vi "Station jsObject Array.vi"(6 "Stations Instruments (none)":cluster{"Instruments":T1[]}[](array[cluster]), 8 "error in (no error)":errorcluster, 9 "Stations (empty)":T2[](array[typedef]), 10 "Stations jsObject Array Name (\"STATIONS\")":string="STATIONS", 11 "Previous String (\"\")":string) -> (0 "error out":errorcluster, 2 "Stations jsObject Array":string, 3 "Station jsObject Definition":string)   [LabVIEW 2011]
uses:
  Station Record.ctl
  Instruments/Instrument Record.ctl
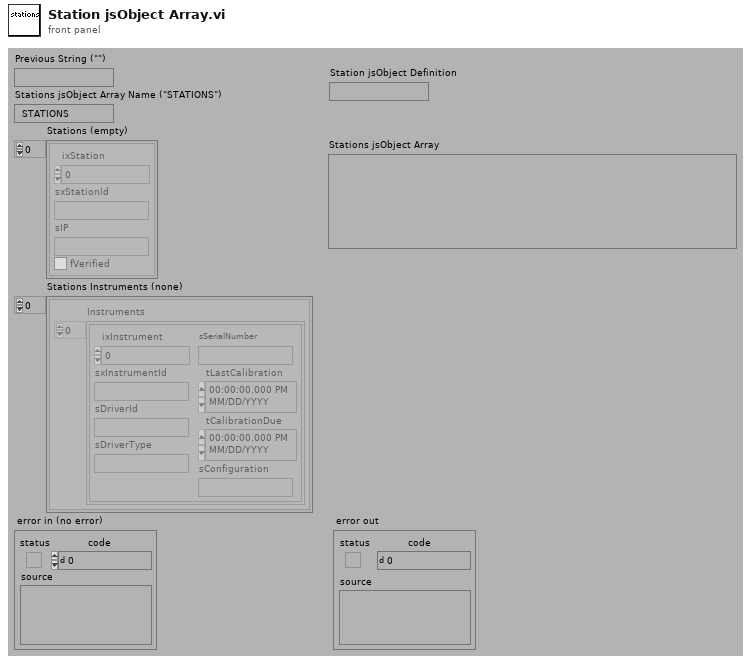
[diagram p1: front panel]
types:
  T1 = typedef "Instrument Record.ctl" = cluster{"ixInstrument":i32, "sxInstrumentId":string, "sDriverId":string, "sDriverType":string, "sSerialNumber":string, "tLastCalibration":timestamp, "tCalibrationDue":timestamp, "sConfiguration":string}
  T2 = typedef "Station Record.ctl" = cluster{"ixStation":i32, "sxStationId":string, "sIP":string, "fVerified":bool}
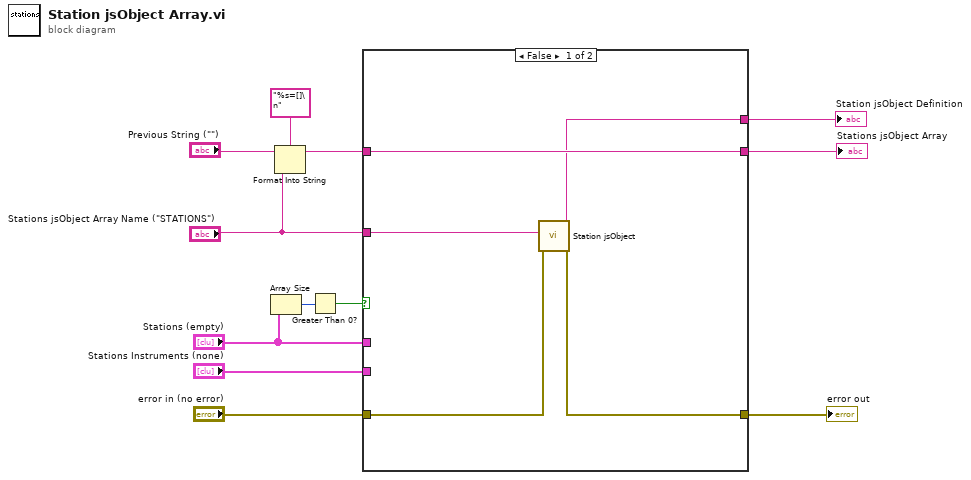
[diagram p0: block diagram]
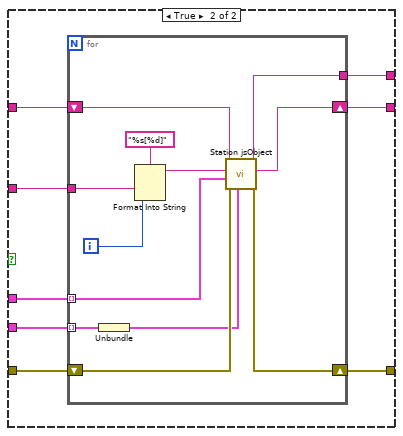
[diagram p2: hidden frame]
diagram:
  n1 = Array Size(array="Stations (empty)") -> (size(s)=w10:i32)
  n2 = Format Into String(format string="%s=[]\n", initial string="Previous String (\"\")", "Stations jsObject Array Name (\"STATIONS\")") -> (resulting string=w11:string)  [unwired: 1 in, 1 out]
  n3 = Greater Than 0?(x=w10) -> (x > 0?=w9:bool)
  n4 = case shown="False" w9 {
    tunnel: w11 -> [w17 w25]
    tunnel: "error in (no error)" -> [w16 w24]
    tunnel: [w17 w23] -> w3
    tunnel: [w15 w22] -> w2
    tunnel: "Stations jsObject Array Name (\"STATIONS\")" -> [w14 w21]
    tunnel: [w13 w20] -> w4
    tunnel: "Stations (empty)" -> [_ w19]
    tunnel: "Stations Instruments (none)" -> [_ w18]
    frame False {
      n5 = call "Station jsObject.vi"("error in (no error)"=w16, "Station jsObject Name (\"\")"=w14) -> ("error out"=w15:errorcluster, "Station jsObject Definition"=w13:string)  [unwired: 3 in, 5 out]
    }
    frame True {
      n6 = for {
        tunnel: w19 -> [w31] mode=indexing
        shift-right: [w30] -> w23
        shift-left: w25 -> [w28]
        shift-right: [w33] -> w22
        shift-left: w24 -> [w34]
        tunnel: w21 -> [w36]
        tunnel: [w29] -> w20
        tunnel: w18 -> [w27] mode=indexing
        i -> [w35]
        n7 = Unbundle(w27) -> ("Instruments"=w26:T1[])
        n8 = Format Into String(format string="%s[%d]", w36, w35) -> (resulting string=w32:string)  [unwired: 2 in, 1 out]
        n9 = call "Station jsObject.vi"("Station Instruments (none)"=w26, "error in (no error)"=w34, "Station Record (empty)"=w31, "Station jsObject Name (\"\")"=w32, "Previous String (\"\")"=w28) -> ("error out"=w33:errorcluster, "Station jsObject"=w30:string, "Station jsObject Definition"=w29:string)  [unwired: 4 out]
      }
    }
  }
  "Stations jsObject Array" <- w3
  "error out" <- w2
  "Station jsObject Definition" <- w4
